vi "Configure Gain.vi"(8 "error in (no error)":errorcluster, 10 "gain":u16(ring) items=["1", "3", "5", "7"], 11 "TroSpec in":refnum<class "PL ISTEQ TroSpec.lvclass">) -> (0 "error out":errorcluster, 3 "TroSpec out":refnum<class "PL ISTEQ TroSpec.lvclass">)   [LabVIEW 2015, in "PL ISTEQ TroSpec.lvclass"]
doc: "Configures CCD gain."
uses:
  PL ISTEQ TroSpec.lvclass
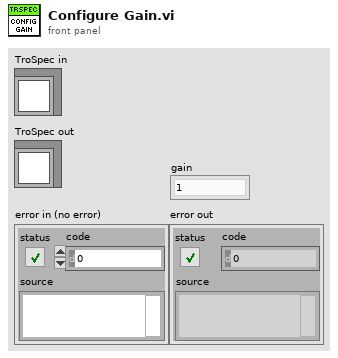
[diagram p1: front panel]
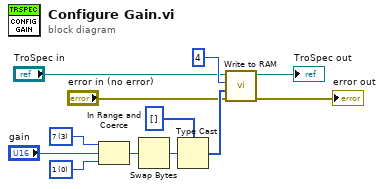
[diagram p0: block diagram]
diagram:
  w2 = u16 3 items=["1", "3", "5", "7"] ("gain")
  w3 = u16 0 items=["1", "3", "5", "7"] ("gain")
  n1 = In Range and Coerce(upper limit=w2, x="gain", lower limit=w3) -> (coerced(x)=w4:u16)  [unwired: 1 out]
  n2 = Swap Bytes(anything=w4) -> (byte swapped=w5:u16)
  n3 = Type Cast(type=u8[] [] ("data"), x=w5) -> (*(type *) &x=w12:u8[])
  n4 = call "Write to RAM.vi"("error in (no error)"="error in (no error)", "data"=w12, "address"=u16 4, "TroSpec in"="TroSpec in") -> ("error out"=→"error out":errorcluster, "TroSpec out"=→"TroSpec out":refnum<class "PL ISTEQ TroSpec.lvclass">)  [unwired: 6 in]
